vi "read_book_notifier.vi"(8 "error in (no error)":errorcluster, 9 "timeout in ms (-1)":i32=-1, 11 "client in":refnum<class "client.lvclass">) -> (0 "error out":errorcluster, 2 "book contents":string, 3 "client out":refnum<class "client.lvclass">)   [LabVIEW 2020, in "client.lvclass"]
uses:
  client.lvclass
  client.lvclass/client.ctl
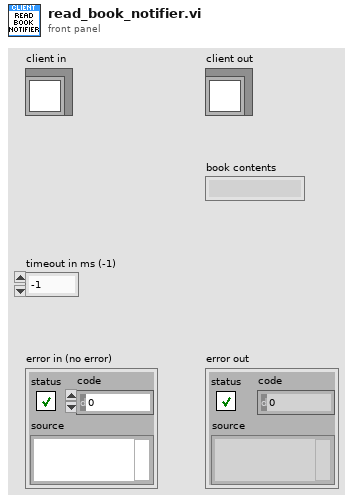
[diagram p1: front panel]
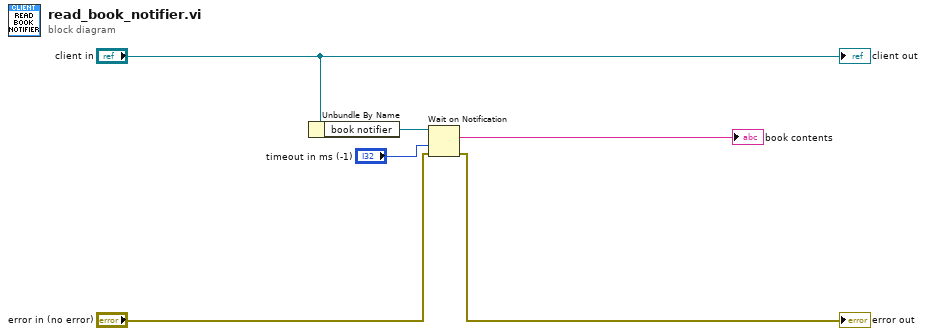
[diagram p0: block diagram]
diagram:
  n1 = Unbundle By Name("client in") -> ("book notifier"=w5:refnum<notifier>)
  n2 = Wait on Notification(notifier=w5, timeout in ms (-1)="timeout in ms (-1)", error in (no error)="error in (no error)") -> (notification=→"book contents":string, error out=→"error out":errorcluster)  [unwired: 1 in, 2 out]
  "client out" <- "client in"
